vi "Create Data Directory.vi"(8 "error in (no error)":errorcluster, 11 "Folder Name":T1) -> (0 "error out":errorcluster, 3 "file path":path)   [LabVIEW 2026]
uses:
  Controls/Folder Name.ctl
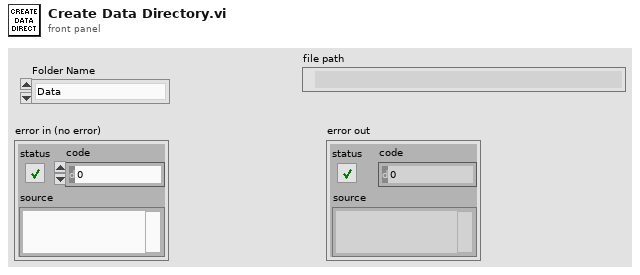
[diagram p1: front panel]
types:
  T1 = typedef "Folder Name.ctl" = enum16{"Data", "TDMS"}
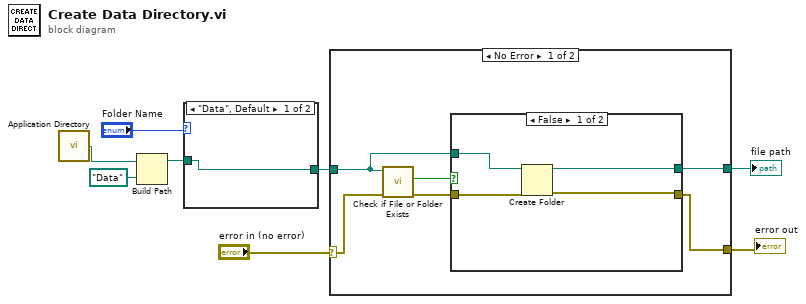
[diagram p0: block diagram]
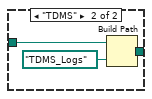
[diagram p2: hidden frame]
diagram:
  n1 = call <vilib>:"Application Directory.vi"() -> ("Application Directory"=w8:path)
  n2 = Build Path(base path=w8, name or relative path=path "Data") -> (appended path=w3:path)
  n3 = case shown="\"Data\", Default" "Folder Name" {
    tunnel: w3 -> [w9 w11]
    tunnel: [w9 w10] -> w2
    frame "Data", Default {
    }
    frame "TDMS" {
      n4 = Build Path(base path=w11, name or relative path=path "TDMS_Logs") -> (appended path=w10:path)
    }
  }
  n5 = case shown="No Error" "error in (no error)" {
    selector: "error in (no error)" -> [w13 w26]
    tunnel: w2 -> [w17 w25]
    tunnel: [w15 w25] -> w6
    tunnel: [w14 w26] -> w4
    frame No Error {
      n6 = call <vilib>:"Check if File or Folder Exists.vi"("error in (no error)"=w13, "path"=w17) -> ("error out"=w16:errorcluster, "file or folder exists?"=w18:bool)  [unwired: 7 in, 1 out]
      n7 = case shown="False" w18 {
        tunnel: w17 -> [w22 w24]
        tunnel: w16 -> [w21 w23]
        tunnel: [w20 w24] -> w15
        tunnel: [w19 w23] -> w14
        frame False {
          n8 = Create Folder(path (use dialog)=w22, error in=w21) -> (created path=w20:path, error out=w19:errorcluster)  [unwired: 1 in, 1 out]
        }
        frame True {
        }
      }
    }
    frame Error {
    }
  }
  "file path" <- w6
  "error out" <- w4
